vi "GCD of array.vi"(11 "Array":u32[](array[numeric])) -> (1 "Divisors":u32[](array[numeric]), 3 "GCD":u32)   [LabVIEW 2020]
doc: "Calculates Greatest Common Divisor. Use naive and slow algorithm. Divisors array is input array divided by GCD."
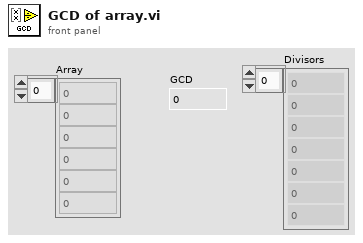
[diagram p1: front panel]
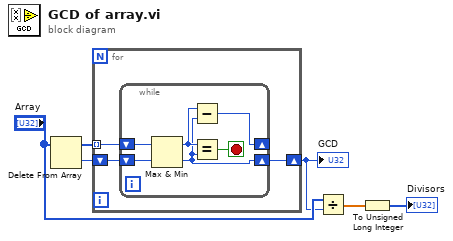
[diagram p0: block diagram]
diagram:
  n1 = Delete From Array(array="Array") -> (deleted portion=w5:u32, array with subset deleted=w6:u32[])  [unwired: 2 in]
  n2 = for {
    tunnel: w6 -> [w9] mode=indexing
    shift-right: [w7] -> w3
    shift-left: w5 -> [w8]
    n3 = while {
      shift-right: [w11] -> w7
      shift-left: w8 -> [w14]
      shift-right: [w13] -> _
      shift-left: w9 -> [w15]
      stop <- w10 stop-if-true
      n4 = Max & Min(x=w15, y=w14) -> (max(x,y)=w12:u32, min(x,y)=w11:u32)
      n5 = Subtract(x=w12, y=w11) -> (x-y=w13:u32)
      n6 = Equal?(x=w12, y=w11) -> (x = y?=w10:bool)
    }
  }
  "GCD" <- w3
  n7 = Divide(x="Array", y=w3) -> (x/y=w2:dbl[])
  n8 = To Unsigned Long Integer(number=w2) -> (unsigned 32bit integer=→"Divisors":u32[])
